vi "EvaluateLcOutputs.vi"(8 "error in (no error)":errorcluster) -> (0 "error out":errorcluster)   [LabVIEW 2019, in "AutoMode.lvlib"]
uses:
  AutoMode.lvlib
panel:
  in  "Offsets":dbl[](array[numeric])
  in  "Data In":dbl[][](array[numeric])
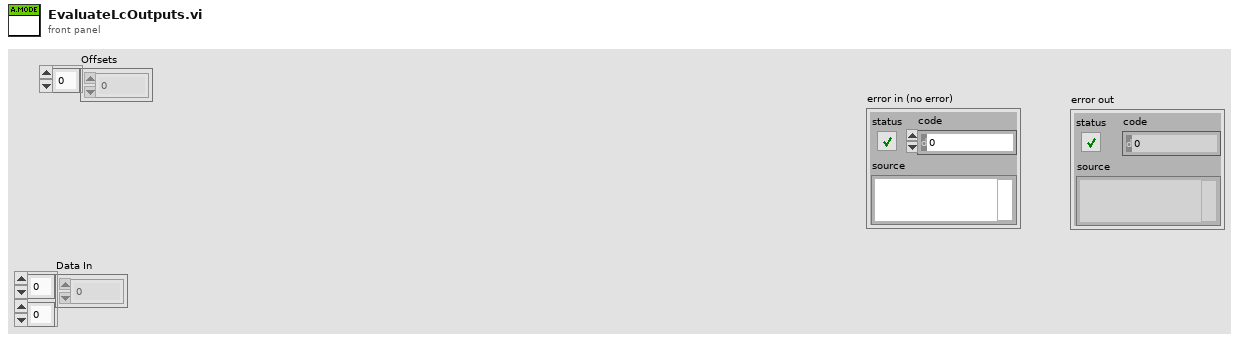
[diagram p1: front panel]
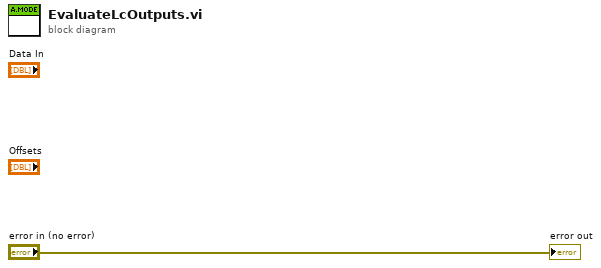
[diagram p0: block diagram]
diagram:
  "error out" <- "error in (no error)"
